vi "CAN_HV_subvi_set_2012.vi"(2 "Voltage":dbl[](array[numeric]), 3 "Power on/off":bool[](array[boolean]), 4 "IP adress HV2":string="0_0_0", 5 "IP adress HV1":string="1_0_0") -> (0 "error out":errorcluster, 1 "handle":i32)   [LabVIEW 2012]
uses:
  Program Files/CAEN/HV/CAENHVWrapper/labview/CAENHVWrapper/CAENHVWrapper.lvlib
panel:
  out "IP adress used":string
  # "Power on/off"
  # "Voltage"
  # "Channel 0"
  # "Channel 1"
  # "Channel 2"
  # "Channel 3"
  # "Channel 4"
  # "Channel 5"
  # "Channel 6"
  # "Channel 7"
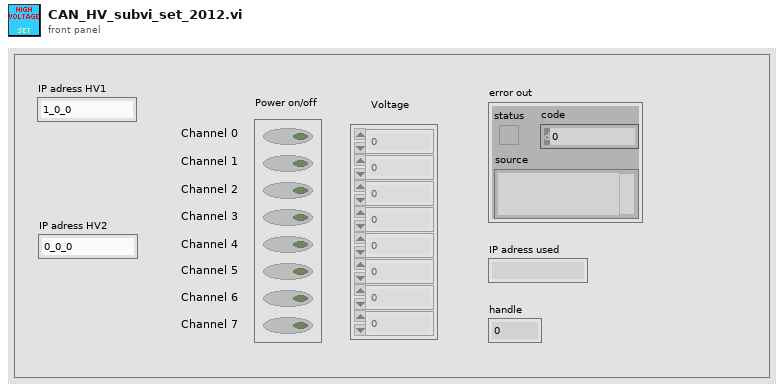
[diagram p1: front panel]
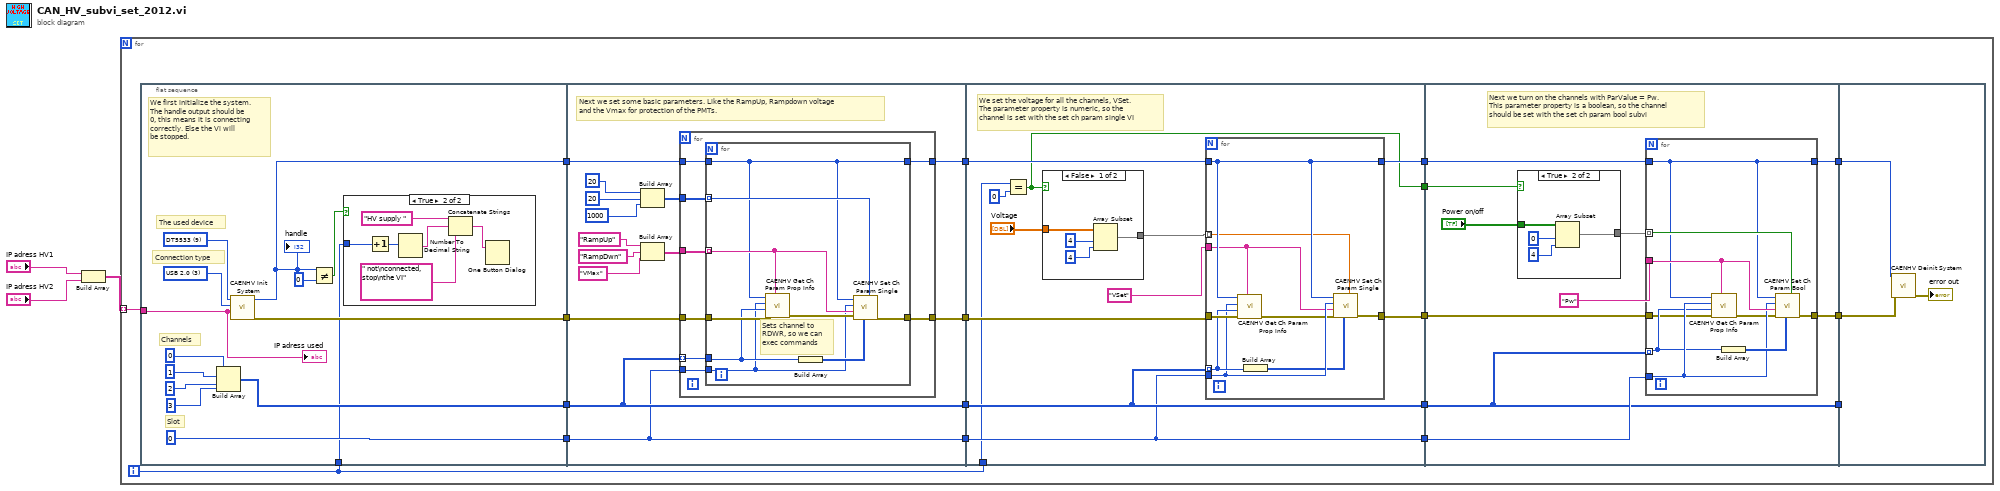
[diagram p0: block diagram]
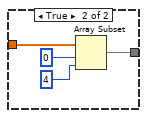
[diagram p3: hidden frame]
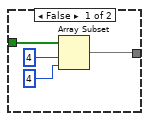
[diagram p4: hidden frame]
diagram:
  n1 = Build Array("IP adress HV1", "IP adress HV2") -> (w1:string[])
  n2 = for {
    tunnel: w1 -> [w9] mode=indexing
    i -> [w4]
    n3 = flat-sequence {
      tunnel: [w33] -> w21
      tunnel: [w29] -> w20
      tunnel: [w30] -> w19
      tunnel: [0] -> w18
      tunnel: w9 -> [w28]
      tunnel: w4 -> [w22]
      tunnel: w21 -> [w53]
      tunnel: w20 -> [w55]
      tunnel: [w54] -> w17
      tunnel: w19 -> [w47]
      tunnel: w18 -> [w46]
      tunnel: [w47] -> w16
      tunnel: [w46] -> w15
      tunnel: [w52] -> w14
      tunnel: w17 -> [w84]
      tunnel: [w83] -> w13
      tunnel: [w80] -> w12
      tunnel: [w82] -> w11
      tunnel: [w81] -> w10
      tunnel: w16 -> [w81]
      tunnel: w15 -> [w80]
      tunnel: w14 -> [w79]
      tunnel: [w75] -> w8
      tunnel: w4 -> [w74]
      tunnel: w13 -> [w110]
      tunnel: w12 -> [w105]
      tunnel: w11 -> [w109]
      tunnel: w10 -> [w104]
      tunnel: w8 -> [w108]
      tunnel: [w107] -> w7
      tunnel: [w106] -> w6
      tunnel: [w104] -> w5
      tunnel: w7 -> [w130]
      tunnel: w6 -> [w129]
      tunnel: w5 -> [_]
      frame #0 {
        w35 = 3 items=["TCP/IP"=0, "HS CAENET"=2, "USB 2.0"=3, "CONET Optical Link"=4, "USB VCP"=5] ("LinkType")
        w34 = u32 9 items=["SY1527", "SY2527", "SY4527", "SY5527", "N568", "V65XX", "N1470", "V8100", "N568E", "DT5533"] ("system")
        # "Connection type"
        # "The used device"
        # "Slot"
        # "Channels"
        # "We first initialize the system.\nThe handle output should be\n0, this means it is connecting\ncorrectly. Else the Vi will\nbe stopped."
        n4 = Build Array(0, 1, 2, 3) -> (w30:i32[])
        n5 = call "CAENHV Init System.vi"("Arg"=w28, "LinkType"=w35, "system"=w34) -> ("error out"=w33:errorcluster, "handle"=w29:i32)  [unwired: 7 in]
        "handle" <- w29
        n6 = Not Equal?(x=w29, y=0) -> (x != y?=w31:bool)
        n7 = case shown="True" w31 {
          tunnel: w22 -> [_ w41]
          frame False {
          }
          frame True {
            n8 = Increment(x=w41) -> (x+1=w40:i32)
            n9 = Number To Decimal String(number=w40) -> (decimal integer string=w38:string)  [unwired: 1 in]
            n10 = Concatenate Strings("HV supply ", w38, " not\nconnected, stop\nthe VI" ("message")) -> (w36:string)
            n11 = One Button Dialog(message=w36) -> ()  [unwired: 1 in, 1 out]
          }
        }
        "IP adress used" <- w28
      }
      frame #1 {
        # "Next we set some basic parameters. Like the RampUp, Rampdown voltage \nand the Vmax for protection of the PMTs."
        n12 = Build Array(20, 20, 1000) -> (w42:i32[])
        n13 = Build Array("RampUp", "RampDwn", "VMax") -> (w48:string[])
        n14 = for {
          tunnel: w55 -> [w58]
          tunnel: [w56] -> w54
          tunnel: w53 -> [w63]
          tunnel: [w62] -> w52
          tunnel: w48 -> [w61]
          tunnel: w47 -> [w60] mode=indexing
          tunnel: w46 -> [w59]
          tunnel: w42 -> [w57]
          n15 = for {
            tunnel: w63 -> [w72]
            tunnel: [w70] -> w62
            tunnel: w61 -> [w68] mode=indexing
            tunnel: w60 -> [w67]
            tunnel: w59 -> [w66]
            tunnel: w58 -> [w64]
            tunnel: w57 -> [w65] mode=indexing
            tunnel: [w64] -> w56
            # "Sets channel to RDWR, so we can exec commands"
            n16 = call "CAENHV Get Ch Param Prop Info.vi"("ParName"=w68, "error in (no error)"=w72, "Ch"=w67, "slot"=w66, "handle"=w64) -> ("error out"=w71:errorcluster)  [unwired: 4 in, 2 out]
            n17 = Build Array(w67) -> (w69:i32[])
            n18 = call "CAENHV Set Ch Param Single.vi"("ParValue"=w65, "ChList"=w69, "error in (no error)"=w71, "ParName"=w68, "slot"=w66, "handle"=w64) -> ("error out"=w70:errorcluster)  [unwired: 5 in]
          }
        }
      }
      frame #2 {
        # "We set the voltage for all the channels, VSet.\nThe parameter property is numeric, so the\nchannel is set with the set ch param single VI"
        n19 = Equal?(x=w74, y=0) -> (x = y?=w75:bool)
        n20 = case shown="False" w75 {
          tunnel: [w85 w90] -> w77
          tunnel: "Voltage" -> [w86 w89]
          frame False {
            n21 = Array Subset(array=w86, index=4, length=4) -> (w85:dbl[])
          }
          frame True {
            n22 = Array Subset(array=w89, index=0, length=4) -> (w90:dbl[])
          }
        }
        n23 = for {
          tunnel: "VSet" ("Setvoltage") -> [w97]
          tunnel: w79 -> [w101]
          tunnel: w81 -> [w100] mode=indexing
          tunnel: w80 -> [w98]
          tunnel: w84 -> [w99]
          tunnel: [w99] -> w83
          tunnel: [w96] -> w82
          tunnel: w77 -> [w95] mode=indexing
          n24 = call "CAENHV Get Ch Param Prop Info.vi"("ParName"=w97, "error in (no error)"=w101, "Ch"=w100, "slot"=w98, "handle"=w99) -> ("error out"=w93:errorcluster)  [unwired: 4 in, 2 out]
          n25 = Build Array(w100) -> (w94:i32[])
          n26 = call "CAENHV Set Ch Param Single.vi"("ParValue"=w95, "ChList"=w94, "error in (no error)"=w93, "ParName"=w97, "slot"=w98, "handle"=w99) -> ("error out"=w96:errorcluster)  [unwired: 5 in]
        }
      }
      frame #3 {
        # "Next we turn on the channels with ParValue = Pw. \nThis parameter property is a boolean, so the channel\nshould be set with the set ch param bool subvi"
        n27 = case shown="True" w108 {
          tunnel: [w112 w117] -> w103
          tunnel: "Power on/off" -> [w113 w116]
          frame False {
            n28 = Array Subset(array=w113, index=4, length=4) -> (w112:bool[])
          }
          frame True {
            n29 = Array Subset(array=w116, index=0, length=4) -> (w117:bool[])
          }
        }
        n30 = for {
          tunnel: w103 -> [w128] mode=indexing
          tunnel: [w127] -> w106
          tunnel: "Pw" ("ParName") -> [w126]
          tunnel: w110 -> [w124]
          tunnel: [w124] -> w107
          tunnel: w105 -> [w123]
          tunnel: w104 -> [w122] mode=indexing
          tunnel: w109 -> [w121]
          n31 = call "CAENHV Get Ch Param Prop Info.vi"("ParName"=w126, "error in (no error)"=w121, "Ch"=w122, "slot"=w123, "handle"=w124) -> ("error out"=w120:errorcluster)  [unwired: 4 in, 2 out]
          n32 = Build Array(w122) -> (w125:i32[])
          n33 = call "CAENHV Set Ch Param Bool.vi"("ParValue"=w128, "ChList"=w125, "error in (no error)"=w120, "ParName"=w126, "slot"=w123, "handle"=w124) -> ("error out"=w127:errorcluster)  [unwired: 5 in]
        }
      }
      frame #4 {
        n34 = call "CAENHV Deinit System.vi"("error in (no error)"=w129, "handle"=w130) -> ("error out"=→"error out":errorcluster)  [unwired: 9 in]
      }
    }
  }
